vi "SMTP Email Send Message.vi"(5 "sender":string, 7 "server":string, 8 "error in (no error)":errorcluster, 9 "message":string, 10 "subject":string, 11 "recipients":string[](array[string])) -> (0 "error out":errorcluster)   [LabVIEW 2013, in "ACNET Monitor.lvlib"]
uses:
  <vilib>/smtpClient/Set Message Text.vi
  ACNET Monitor.lvlib
  <vilib>/smtpClient/LabVIEWSMTPClient.lvlib
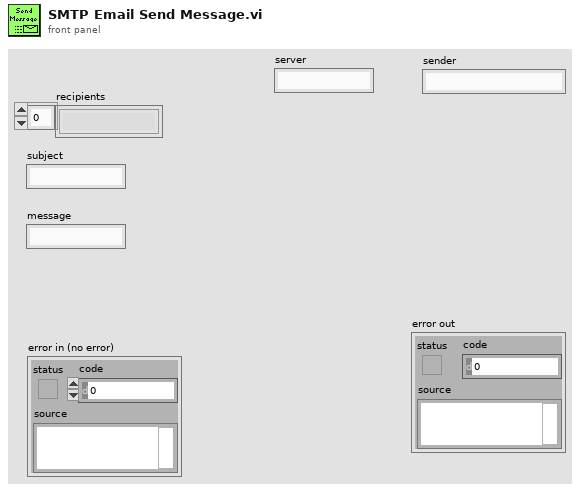
[diagram p1: front panel]
types:
  T1 = typedef "LabVIEWSMTPClient.lvlib/SmtpClientHandle.ctl" = refnum<k1>
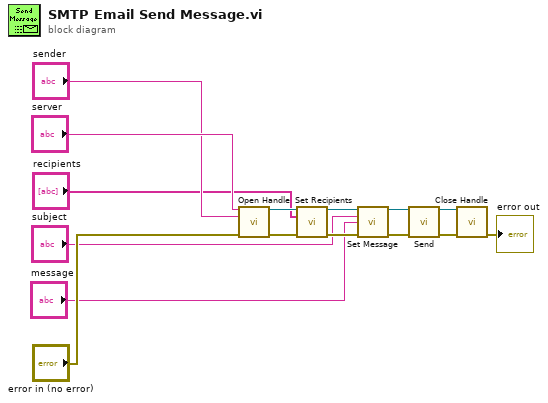
[diagram p0: block diagram]
diagram:
  n1 = call <vilib>:"Open Handle.vi"("server address"="server", "from"="sender", "error in (no error)"="error in (no error)") -> ("handle out"=w12:T1, "error out"=w11:errorcluster)  [unwired: 11 in]
  n2 = call <vilib>:"Set Recipients.vi"("handle in"=w12, "to"="recipients", "error in (no error)"=w11) -> ("handle out"=w9:T1, "error out"=w8:errorcluster)  [unwired: 11 in]
  n3 = call-poly <vilib>:"Set Message.vi"("handle in"=w9, "subject"="subject", "plain text message"="message", "error in (no error)"=w8) -> ("handle out"=w4:T1, "error out"=w5:errorcluster)  [unwired: 10 in]
  n4 = call <vilib>:"Send.vi"("handle in"=w4, "error in (no error)"=w5) -> ("handle out"=w3:T1, "error out"=w2:errorcluster)  [unwired: 11 in, 1 out]
  n5 = call <vilib>:"Close Handle.vi"("handle in"=w3, "error in (no error)"=w2) -> ("error out"=→"error out":errorcluster)  [unwired: 12 in, 1 out]
